vi "(SubVI)I2C_Log_Append LF.vi"(5 "Log Ref":refnum<vi>, 10 "error in (no error)":errorcluster caption="에러 입력(에러 없음)", 11 "Str to Append before LF":string) -> (2 "error out":errorcluster caption="에러 출력")   [LabVIEW 2020]
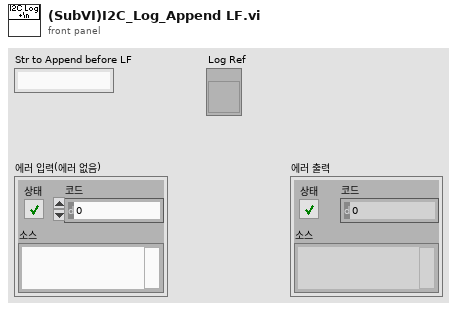
[diagram p1: front panel]
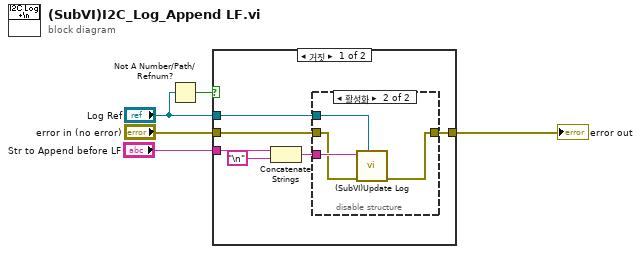
[diagram p0: block diagram]
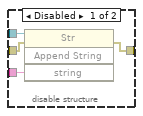
[diagram p2: hidden frame]
diagram:
  n1 = Not A Number/Path/Refnum?(number/path/refnum="Log Ref") -> (NaN/Path/Refnum?=w4:bool)
  n2 = case shown="거짓" w4 {
    tunnel: "Log Ref" -> [w11 _]
    tunnel: "error in (no error)" -> [w10 w20]
    tunnel: [w9 w20] -> w2
    tunnel: "Str to Append before LF" -> [w7 _]
    frame False {
      n3 = Concatenate Strings(w7, "\n" ("문자열")) -> (w6:string)
      n4 = disable-structure shown="활성화" {
        disable-tunnel: w11 -> [w15 w18]
        disable-tunnel: w10 -> [w14 w17]
        disable-tunnel: [w13 w16] -> w9
        disable-tunnel: w6 -> [w12 w19]
        frame Disabled {
          n5 = invoke class="Str" method="Append String"(reference=w15, error in=w14, "string"=w12) -> (error out=w13:errorcluster)  [unwired: 1 in, 3 out]
        }
        frame Enabled {
          n6 = call "(SubVI)Update Log.vi"("Log Ref"=w18, "error in (no error)"=w17, "Log"=w19) -> ("error out"=w16:errorcluster)  [unwired: 7 in, 1 out]
        }
      }
    }
    frame True {
    }
  }
  "error out" <- w2
